vi "get active SPAN indices.vi"(8 "error in (no error)":errorcluster caption="Fehler (Eingang, kein Fehler)", 10 "max active SPAN Idx in":i32, 11 "SpanInletClusterArray in":T1[](array[typedef]) {"zusätzliche Zeitdauer Erster Punkt" min=30 step=1 format="%#_5g"; "Zeitdauer Stufen" format="%#_5g"; "Max Fehler" format="%#_5g"; "Anzahl Stufen" format="%#_5g"; "Komponenten"."Komponente 5"."Komponente:" items=["NO (350,3000) LP 191C", "NO2 (150) LP 191C (1of2)", "NO2 (2000) LP 191C (2of2)", "N2O (300) LP 191C (1of2)", "NH3 (300) LP 191C (1of2)", "NH3 (900,3000) LP 191C (2of2)", "HNCO (400) 191C", "H2O% (30) LP 191C", "Formaldehyde (70,500) LP 191C", "CO2 low% (4) LP 191C (2of2)", "CO2% (20) LP 191C (1of2)", "CO (700) LP 191C (1of3)", "CO% (1) LP 191C (2of3)", "Propylene (1000) LP 191C", "Aromatic HC C7 (500) LP 191C", "Ethylene (1000) LP 191C", "CH4 (250) LP 191C (1of2)", "CH4 (5000) LP 191C (2of2)", "Ethane (1000) LP 191C", "Acetylene (1000) LP 191C", "HNO2 (20) 191C", "MeOH (1000) 191C", "CO% (10) LP 191C (3of3)", "Formic Acid (100) 191C", "SO2 (500) LP 191C", "Acetaldehyde (1000) LP 191C", "COS (100) LP 191C", "1,3 butadiene (100) LP 191C", "Oil as Octane (200) LP 191C", "N2O (1000) LP 191C (2of2)", "Propane (200) LP 191C", "NO2 autorange (2000)", "CO autorange (100000)", "CH4 autorange (5000)", "NH3 autorange (3000)", "Temp. Gascell", "Pressure Gascell", "sBeam@2500"]; "Komponenten"."Komponente 5"."Konzentration IST" format="%#.4f"; "Komponenten"."Komponente 5"."Genauigkeit" format="%#.1f"; "Komponenten"."Komponente 4"."Komponente:" items=["NO (350,3000) LP 191C", "NO2 (150) LP 191C (1of2)", "NO2 (2000) LP 191C (2of2)", "N2O (300) LP 191C (1of2)", "NH3 (300) LP 191C (1of2)", "NH3 (900,3000) LP 191C (2of2)", "HNCO (400) 191C", "H2O% (30) LP 191C", "Formaldehyde (70,500) LP 191C", "CO2 low% (4) LP 191C (2of2)", "CO2% (20) LP 191C (1of2)", "CO (700) LP 191C (1of3)", "CO% (1) LP 191C (2of3)", "Propylene (1000) LP 191C", "Aromatic HC C7 (500) LP 191C", "Ethylene (1000) LP 191C", "CH4 (250) LP 191C (1of2)", "CH4 (5000) LP 191C (2of2)", "Ethane (1000) LP 191C", "Acetylene (1000) LP 191C", "HNO2 (20) 191C", "MeOH (1000) 191C", "CO% (10) LP 191C (3of3)", "Formic Acid (100) 191C", "SO2 (500) LP 191C", "Acetaldehyde (1000) LP 191C", "COS (100) LP 191C", "1,3 butadiene (100) LP 191C", "Oil as Octane (200) LP 191C", "N2O (1000) LP 191C (2of2)", "Propane (200) LP 191C", "NO2 autorange (2000)", "CO autorange (100000)", "CH4 autorange (5000)", "NH3 autorange (3000)", "Temp. Gascell", "Pressure Gascell", "sBeam@2500"]; "Komponenten"."Komponente 4"."Konzentration IST" format="%#.4f"; "Komponenten"."Komponente 4"."Genauigkeit" format="%#.1f"; "Komponenten"."Komponente 3"."Komponente:" items=["NO (350,3000) LP 191C", "NO2 (150) LP 191C (1of2)", "NO2 (2000) LP 191C (2of2)", "N2O (300) LP 191C (1of2)", "NH3 (300) LP 191C (1of2)", "NH3 (900,3000) LP 191C (2of2)", "HNCO (400) 191C", "H2O% (30) LP 191C", "Formaldehyde (70,500) LP 191C", "CO2 low% (4) LP 191C (2of2)", "CO2% (20) LP 191C (1of2)", "CO (700) LP 191C (1of3)", "CO% (1) LP 191C (2of3)", "Propylene (1000) LP 191C", "Aromatic HC C7 (500) LP 191C", "Ethylene (1000) LP 191C", "CH4 (250) LP 191C (1of2)", "CH4 (5000) LP 191C (2of2)", "Ethane (1000) LP 191C", "Acetylene (1000) LP 191C", "HNO2 (20) 191C", "MeOH (1000) 191C", "CO% (10) LP 191C (3of3)", "Formic Acid (100) 191C", "SO2 (500) LP 191C", "Acetaldehyde (1000) LP 191C", "COS (100) LP 191C", "1,3 butadiene (100) LP 191C", "Oil as Octane (200) LP 191C", "N2O (1000) LP 191C (2of2)", "Propane (200) LP 191C", "NO2 autorange (2000)", "CO autorange (100000)", "CH4 autorange (5000)", "NH3 autorange (3000)", "Temp. Gascell", "Pressure Gascell", "sBeam@2500"]; "Komponenten"."Komponente 3"."Konzentration IST" format="%#.4f"; "Komponenten"."Komponente 3"."Genauigkeit" format="%#.1f"; "Komponenten"."Komponente 2"."Komponente:" items=["NO (350,3000) LP 191C", "NO2 (150) LP 191C (1of2)", "NO2 (2000) LP 191C (2of2)", "N2O (300) LP 191C (1of2)", "NH3 (300) LP 191C (1of2)", "NH3 (900,3000) LP 191C (2of2)", "HNCO (400) 191C", "H2O% (30) LP 191C", "Formaldehyde (70,500) LP 191C", "CO2 low% (4) LP 191C (2of2)", "CO2% (20) LP 191C (1of2)", "CO (700) LP 191C (1of3)", "CO% (1) LP 191C (2of3)", "Propylene (1000) LP 191C", "Aromatic HC C7 (500) LP 191C", "Ethylene (1000) LP 191C", "CH4 (250) LP 191C (1of2)", "CH4 (5000) LP 191C (2of2)", "Ethane (1000) LP 191C", "Acetylene (1000) LP 191C", "HNO2 (20) 191C", "MeOH (1000) 191C", "CO% (10) LP 191C (3of3)", "Formic Acid (100) 191C", "SO2 (500) LP 191C", "Acetaldehyde (1000) LP 191C", "COS (100) LP 191C", "1,3 butadiene (100) LP 191C", "Oil as Octane (200) LP 191C", "N2O (1000) LP 191C (2of2)", "Propane (200) LP 191C", "NO2 autorange (2000)", "CO autorange (100000)", "CH4 autorange (5000)", "NH3 autorange (3000)", "Temp. Gascell", "Pressure Gascell", "sBeam@2500"]; "Komponenten"."Komponente 2"."Konzentration IST" format="%#.4f"; "Komponenten"."Komponente 2"."Genauigkeit" format="%#.1f"; "Komponenten"."Komponente 1"."Komponente:" items=["NO (350,3000) LP 191C", "NO2 (150) LP 191C (1of2)", "NO2 (2000) LP 191C (2of2)", "N2O (300) LP 191C (1of2)", "NH3 (300) LP 191C (1of2)", "NH3 (900,3000) LP 191C (2of2)", "HNCO (400) 191C", "H2O% (30) LP 191C", "Formaldehyde (70,500) LP 191C", "CO2 low% (4) LP 191C (2of2)", "CO2% (20) LP 191C (1of2)", "CO (700) LP 191C (1of3)", "CO% (1) LP 191C (2of3)", "Propylene (1000) LP 191C", "Aromatic HC C7 (500) LP 191C", "Ethylene (1000) LP 191C", "CH4 (250) LP 191C (1of2)", "CH4 (5000) LP 191C (2of2)", "Ethane (1000) LP 191C", "Acetylene (1000) LP 191C", "HNO2 (20) 191C", "MeOH (1000) 191C", "CO% (10) LP 191C (3of3)", "Formic Acid (100) 191C", "SO2 (500) LP 191C", "Acetaldehyde (1000) LP 191C", "COS (100) LP 191C", "1,3 butadiene (100) LP 191C", "Oil as Octane (200) LP 191C", "N2O (1000) LP 191C (2of2)", "Propane (200) LP 191C", "NO2 autorange (2000)", "CO autorange (100000)", "CH4 autorange (5000)", "NH3 autorange (3000)", "Temp. Gascell", "Pressure Gascell", "sBeam@2500"]; "Komponenten"."Komponente 1"."Konzentration IST" format="%#.4f"; "Komponenten"."Komponente 1"."Genauigkeit" format="%#.1f"; "Ablaufdatum" format="%<%d.%m.%Y>T"; "Gasflasche" items=["----"=10000, "IAG NH3 3000"=0, "IAG NH3 200"=1, "IAG NH3 2000"=2, "IAG MG"=3, "IAG O2"=4]}) -> (0 "error out":errorcluster caption="Fehler (Ausgang)", 2 "Index active SPAN":i32[](array[numeric]), 3 "SpanInletClusterArray out":T1[](array[typedef]) {"zusätzliche Zeitdauer Erster Punkt" min=30 step=1 format="%#_5g"; "Zeitdauer Stufen" format="%#_5g"; "Max Fehler" format="%#_5g"; "Anzahl Stufen" format="%#_5g"; "Komponenten"."Komponente 5"."Komponente:" items=["NO (350,3000) LP 191C", "NO2 (150) LP 191C (1of2)", "NO2 (2000) LP 191C (2of2)", "N2O (300) LP 191C (1of2)", "NH3 (300) LP 191C (1of2)", "NH3 (900,3000) LP 191C (2of2)", "HNCO (400) 191C", "H2O% (30) LP 191C", "Formaldehyde (70,500) LP 191C", "CO2 low% (4) LP 191C (2of2)", "CO2% (20) LP 191C (1of2)", "CO (700) LP 191C (1of3)", "CO% (1) LP 191C (2of3)", "Propylene (1000) LP 191C", "Aromatic HC C7 (500) LP 191C", "Ethylene (1000) LP 191C", "CH4 (250) LP 191C (1of2)", "CH4 (5000) LP 191C (2of2)", "Ethane (1000) LP 191C", "Acetylene (1000) LP 191C", "HNO2 (20) 191C", "MeOH (1000) 191C", "CO% (10) LP 191C (3of3)", "Formic Acid (100) 191C", "SO2 (500) LP 191C", "Acetaldehyde (1000) LP 191C", "COS (100) LP 191C", "1,3 butadiene (100) LP 191C", "Oil as Octane (200) LP 191C", "N2O (1000) LP 191C (2of2)", "Propane (200) LP 191C", "NO2 autorange (2000)", "CO autorange (100000)", "CH4 autorange (5000)", "NH3 autorange (3000)", "Temp. Gascell", "Pressure Gascell", "sBeam@2500"]; "Komponenten"."Komponente 5"."Konzentration IST" format="%#.4f"; "Komponenten"."Komponente 5"."Genauigkeit" format="%#.1f"; "Komponenten"."Komponente 4"."Komponente:" items=["NO (350,3000) LP 191C", "NO2 (150) LP 191C (1of2)", "NO2 (2000) LP 191C (2of2)", "N2O (300) LP 191C (1of2)", "NH3 (300) LP 191C (1of2)", "NH3 (900,3000) LP 191C (2of2)", "HNCO (400) 191C", "H2O% (30) LP 191C", "Formaldehyde (70,500) LP 191C", "CO2 low% (4) LP 191C (2of2)", "CO2% (20) LP 191C (1of2)", "CO (700) LP 191C (1of3)", "CO% (1) LP 191C (2of3)", "Propylene (1000) LP 191C", "Aromatic HC C7 (500) LP 191C", "Ethylene (1000) LP 191C", "CH4 (250) LP 191C (1of2)", "CH4 (5000) LP 191C (2of2)", "Ethane (1000) LP 191C", "Acetylene (1000) LP 191C", "HNO2 (20) 191C", "MeOH (1000) 191C", "CO% (10) LP 191C (3of3)", "Formic Acid (100) 191C", "SO2 (500) LP 191C", "Acetaldehyde (1000) LP 191C", "COS (100) LP 191C", "1,3 butadiene (100) LP 191C", "Oil as Octane (200) LP 191C", "N2O (1000) LP 191C (2of2)", "Propane (200) LP 191C", "NO2 autorange (2000)", "CO autorange (100000)", "CH4 autorange (5000)", "NH3 autorange (3000)", "Temp. Gascell", "Pressure Gascell", "sBeam@2500"]; "Komponenten"."Komponente 4"."Konzentration IST" format="%#.4f"; "Komponenten"."Komponente 4"."Genauigkeit" format="%#.1f"; "Komponenten"."Komponente 3"."Komponente:" items=["NO (350,3000) LP 191C", "NO2 (150) LP 191C (1of2)", "NO2 (2000) LP 191C (2of2)", "N2O (300) LP 191C (1of2)", "NH3 (300) LP 191C (1of2)", "NH3 (900,3000) LP 191C (2of2)", "HNCO (400) 191C", "H2O% (30) LP 191C", "Formaldehyde (70,500) LP 191C", "CO2 low% (4) LP 191C (2of2)", "CO2% (20) LP 191C (1of2)", "CO (700) LP 191C (1of3)", "CO% (1) LP 191C (2of3)", "Propylene (1000) LP 191C", "Aromatic HC C7 (500) LP 191C", "Ethylene (1000) LP 191C", "CH4 (250) LP 191C (1of2)", "CH4 (5000) LP 191C (2of2)", "Ethane (1000) LP 191C", "Acetylene (1000) LP 191C", "HNO2 (20) 191C", "MeOH (1000) 191C", "CO% (10) LP 191C (3of3)", "Formic Acid (100) 191C", "SO2 (500) LP 191C", "Acetaldehyde (1000) LP 191C", "COS (100) LP 191C", "1,3 butadiene (100) LP 191C", "Oil as Octane (200) LP 191C", "N2O (1000) LP 191C (2of2)", "Propane (200) LP 191C", "NO2 autorange (2000)", "CO autorange (100000)", "CH4 autorange (5000)", "NH3 autorange (3000)", "Temp. Gascell", "Pressure Gascell", "sBeam@2500"]; "Komponenten"."Komponente 3"."Konzentration IST" format="%#.4f"; "Komponenten"."Komponente 3"."Genauigkeit" format="%#.1f"; "Komponenten"."Komponente 2"."Komponente:" items=["NO (350,3000) LP 191C", "NO2 (150) LP 191C (1of2)", "NO2 (2000) LP 191C (2of2)", "N2O (300) LP 191C (1of2)", "NH3 (300) LP 191C (1of2)", "NH3 (900,3000) LP 191C (2of2)", "HNCO (400) 191C", "H2O% (30) LP 191C", "Formaldehyde (70,500) LP 191C", "CO2 low% (4) LP 191C (2of2)", "CO2% (20) LP 191C (1of2)", "CO (700) LP 191C (1of3)", "CO% (1) LP 191C (2of3)", "Propylene (1000) LP 191C", "Aromatic HC C7 (500) LP 191C", "Ethylene (1000) LP 191C", "CH4 (250) LP 191C (1of2)", "CH4 (5000) LP 191C (2of2)", "Ethane (1000) LP 191C", "Acetylene (1000) LP 191C", "HNO2 (20) 191C", "MeOH (1000) 191C", "CO% (10) LP 191C (3of3)", "Formic Acid (100) 191C", "SO2 (500) LP 191C", "Acetaldehyde (1000) LP 191C", "COS (100) LP 191C", "1,3 butadiene (100) LP 191C", "Oil as Octane (200) LP 191C", "N2O (1000) LP 191C (2of2)", "Propane (200) LP 191C", "NO2 autorange (2000)", "CO autorange (100000)", "CH4 autorange (5000)", "NH3 autorange (3000)", "Temp. Gascell", "Pressure Gascell", "sBeam@2500"]; "Komponenten"."Komponente 2"."Konzentration IST" format="%#.4f"; "Komponenten"."Komponente 2"."Genauigkeit" format="%#.1f"; "Komponenten"."Komponente 1"."Komponente:" items=["NO (350,3000) LP 191C", "NO2 (150) LP 191C (1of2)", "NO2 (2000) LP 191C (2of2)", "N2O (300) LP 191C (1of2)", "NH3 (300) LP 191C (1of2)", "NH3 (900,3000) LP 191C (2of2)", "HNCO (400) 191C", "H2O% (30) LP 191C", "Formaldehyde (70,500) LP 191C", "CO2 low% (4) LP 191C (2of2)", "CO2% (20) LP 191C (1of2)", "CO (700) LP 191C (1of3)", "CO% (1) LP 191C (2of3)", "Propylene (1000) LP 191C", "Aromatic HC C7 (500) LP 191C", "Ethylene (1000) LP 191C", "CH4 (250) LP 191C (1of2)", "CH4 (5000) LP 191C (2of2)", "Ethane (1000) LP 191C", "Acetylene (1000) LP 191C", "HNO2 (20) 191C", "MeOH (1000) 191C", "CO% (10) LP 191C (3of3)", "Formic Acid (100) 191C", "SO2 (500) LP 191C", "Acetaldehyde (1000) LP 191C", "COS (100) LP 191C", "1,3 butadiene (100) LP 191C", "Oil as Octane (200) LP 191C", "N2O (1000) LP 191C (2of2)", "Propane (200) LP 191C", "NO2 autorange (2000)", "CO autorange (100000)", "CH4 autorange (5000)", "NH3 autorange (3000)", "Temp. Gascell", "Pressure Gascell", "sBeam@2500"]; "Komponenten"."Komponente 1"."Konzentration IST" format="%#.4f"; "Komponenten"."Komponente 1"."Genauigkeit" format="%#.1f"; "Ablaufdatum" format="%<%d.%m.%Y>T"; "Gasflasche" items=["----"=10000, "IAG NH3 3000"=0, "IAG NH3 200"=1, "IAG NH3 2000"=2, "IAG MG"=3, "IAG O2"=4]})   [LabVIEW 2020, in "Linearisierung v2.lvlib" / "SpanEinstellungen.lvlib"]
uses:
  SpanEinstellungen.lvlib
  SpanInletCluster.ctl
  Seiten/System Einstellungen V2/Konfig Gasflasche.ctl
  Seiten/System Einstellungen V2/Analysatoren.ctl
  Seiten/System Einstellungen V2/Gasflasche Auswahl.ctl
  Komponentencluster mit Formel.ctl
  Komponentenauswahl mit Formel.ctl
  Visualisierungs Elemente/String - Eingabefeld.ctl
  Einheit.ctl
  Seiten/System Einstellungen V2/Traegergas.ctl
  Seiten/System Einstellungen V2/System Einstellungen V2.lvlib
panel:
  # "sec"
  # "%"
  # "sec"
  # "Komponente"
  # "Formel"
  # "Konzentration"
  # "Einheit"
  # "Genauigkeit [%]"
  # "sec"
  # "%"
  # "sec"
  # "Komponente"
  # "Formel"
  # "Konzentration"
  # "Einheit"
  # "Genauigkeit [%]"
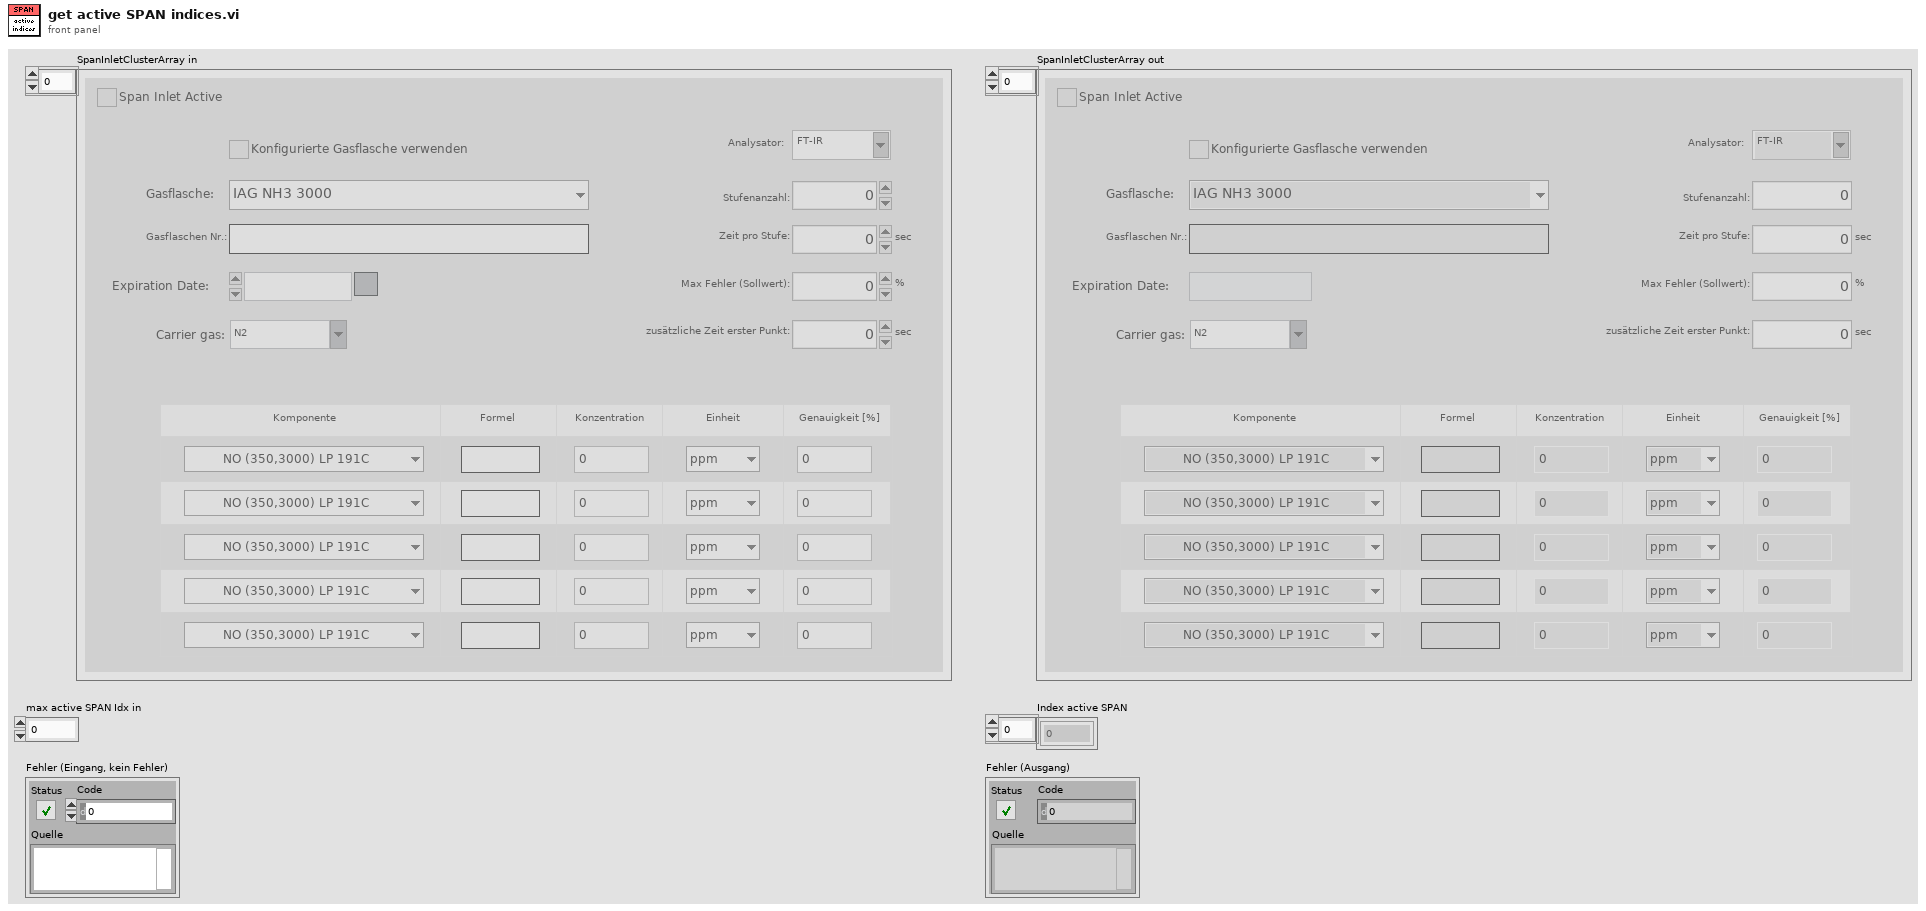
[diagram p1: front panel]
types:
  T1 = typedef "Linearisierung v2.lvlib/SpanEinstellungen.lvlib/SpanInletCluster.ctl" = cluster{"Span Inlet Active":T2, "Analysator":T3, "Konfig Gasflasche":T2, "Gasflasche":T4, "Gasflaschen Nr.:":string, "Ablaufdatum":timestamp, "Komponenten":T5, "Zeitdauer Stufen":sgl, "Max Fehler":sgl, "Anzahl Stufen":sgl, "Trägergas":T9, "zusätzliche Zeitdauer Erster Punkt":sgl}
  T2 = typedef "System Einstellungen V2.lvlib/Konfig Gasflasche.ctl" = bool
  T3 = typedef "System Einstellungen V2.lvlib/Analysatoren.ctl" = string
  T4 = typedef "System Einstellungen V2.lvlib/Gasflasche Auswahl.ctl" = u16
  T5 = typedef "Linearisierung v2.lvlib/SpanEinstellungen.lvlib/Komponentencluster mit Formel.ctl" = cluster{"Komponente 1":T6, "Komponente 2":T6, "Komponente 3":T6, "Komponente 4":T6, "Komponente 5":T6}
  T6 = typedef "Linearisierung v2.lvlib/SpanEinstellungen.lvlib/Komponentenauswahl mit Formel.ctl" = cluster{"Komponente:":u16, "Summenformel":T7, "Konzentration IST":dbl, "Einheit":T8, "Genauigkeit":dbl}
  T7 = typedef "String - Eingabefeld.ctl" = string
  T8 = typedef "Linearisierung v2.lvlib/SpanEinstellungen.lvlib/Einheit.ctl" = enum16{"ppm", "%"}
  T9 = typedef "System Einstellungen V2.lvlib/Traegergas.ctl" = string
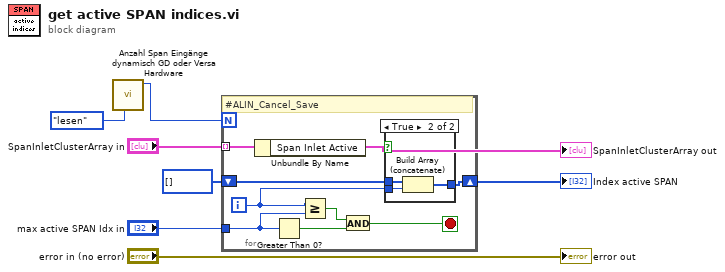
[diagram p0: block diagram]
diagram:
  n1 = call "Anzahl Span Eingänge dynamisch GD oder Versa Hardware.vi"("Aktion"=enum16{"lesen", "schreiben"}."lesen") -> ("Anzahl Span out"=w4:i32)  [unwired: 10 in]
  n2 = for {
    N: w4 -> [_]
    tunnel: "SpanInletClusterArray in" -> [w16] mode=indexing
    shift-right: [w14] -> w2
    shift-left: i32[] [] -> [w13]
    tunnel: "max active SPAN Idx in" -> [w10]
    i -> [w11]
    stop <- w8 stop-if-true
    # "#ALIN_Cancel_Save"
    n3 = Unbundle By Name(w16) -> ("Span Inlet Active"=w15:T2)
    n4 = Greater Than 0?(x=w10) -> (x > 0?=w12:bool)
    n5 = Greater Or Equal?(x=w11, y=w10) -> (x >= y?=w9:bool)
    n6 = And(x=w9, y=w12) -> (x .and. y?=w8:bool)
    n7 = case shown="True" w15 {
      tunnel: w11 -> [_ w20]
      tunnel: [w17 w19] -> w14
      tunnel: w13 -> [w17 w18]
      frame False {
      }
      frame True {
        n8 = Build Array (concatenate)(w18, w20) -> (w19:i32[])
      }
    }
  }
  "Index active SPAN" <- w2
  "SpanInletClusterArray out" <- "SpanInletClusterArray in"
  "error out" <- "error in (no error)"
